vi "Read Voltage.vi"(8 "error in (no error)":errorcluster, 11 "HVPS in":refnum<class "HVPS.lvclass">) -> (0 "error out":errorcluster, 2 "Voltage":sgl, 3 "HVPS out":refnum<class "HVPS.lvclass">)   [LabVIEW 2013, in "HVPS.lvclass"]
uses:
  HVPS.lvclass
  HVPS.lvclass/HVPS.ctl
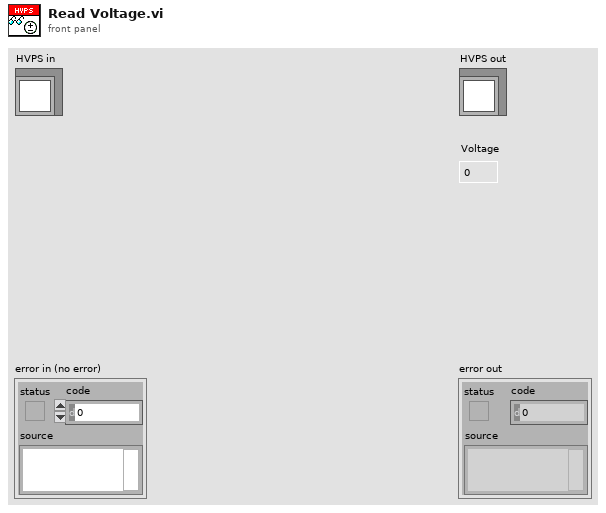
[diagram p1: front panel]
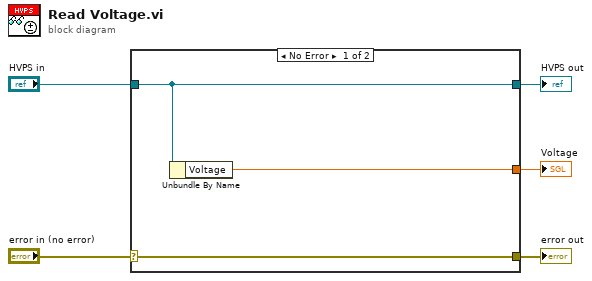
[diagram p0: block diagram]
diagram:
  n1 = case shown="No Error" "error in (no error)" {
    selector: "error in (no error)" -> [w8 w9]
    tunnel: [w8 w9] -> w4
    tunnel: [w7 w10] -> w2
    tunnel: "HVPS in" -> [w7 w10]
    tunnel: [w6 _] -> w1
    frame No Error {
      n2 = Unbundle By Name(w7) -> ("Voltage"=w6:sgl)
    }
    frame Error {
    }
  }
  "error out" <- w4
  "HVPS out" <- w2
  "Voltage" <- w1
